vi "AsyncMessageCore.vi"(6 "Timeout (ms)":i32=-1, 7 "Collect Response?":bool, 8 "error in (no error)":errorcluster, 9 "Payload":string, 10 "Command":string, 11 "GRPCClient in":refnum<class "MicronGRPCClient.lvclass">) -> (0 "error out":errorcluster, 3 "GRPCClient out":refnum<class "MicronGRPCClient.lvclass">)   [LabVIEW 2019, in "MicronGRPCClient.lvclass"]
uses:
  MicronGRPCClient.lvclass
  Generated/MicronGRPCGeneratedClient/RPC Messages/micronGrpc_MessageRequest.ctl
  Typedefs/AsyncMessageRequest.ctl
  Typedefs/gRPCDetails.ctl
  <vilib>/gRPC/LabVIEW gRPC Library/Shared/grpcId.ctl
  MicronGRPCClient.lvclass/MicronGRPCClient.ctl
  <vilib>/SLL Toolkit/SLL Queued State Machine/Queue Driver/Enqueue an Item to Queue.vi
  Generated/MicronGRPCGeneratedClient/MicronGRPCGeneratedClient.lvlib
  <vilib>/gRPC/LabVIEW gRPC Library/grpc-lvsupport-release.lvlib
  <vilib>/SLL Toolkit/SLL Queued State Machine/SLL QSM.lvlib
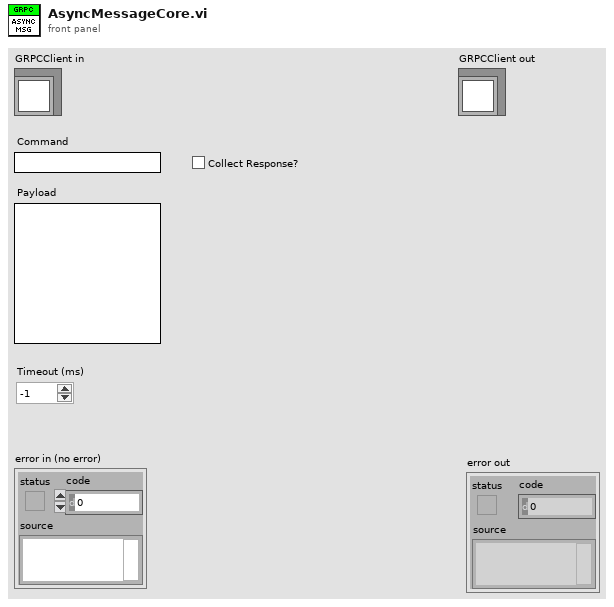
[diagram p1: front panel]
types:
  T1 = typedef "MicronGRPCClient.lvclass/AsyncMessageRequest.ctl" = cluster{"gRPC":T2, "Message":T4, "Timeout (ms)":i32, "Collect Response?":bool}
  T2 = typedef "MicronGRPCClient.lvclass/gRPCDetails.ctl" = cluster{"ID":T3, "PackageName":string, "ServiceName":string, "Simulate?":bool, "ConnectionString":string}
  T3 = typedef "grpc-lvsupport-release.lvlib/grpcId.ctl" = u64
  T4 = typedef "MicronGRPCGeneratedClient.lvlib/micronGrpc_MessageRequest.ctl" = cluster{"command":string, "payload":string}
  T5 = typedef "MicronGRPCClient.lvclass/AsyncCluster.ctl" = cluster{"QueueRef":refnum<queue>, "PackageName":string, "ServiceName":string, "gRPC ID":T3, "Simulate?":bool}
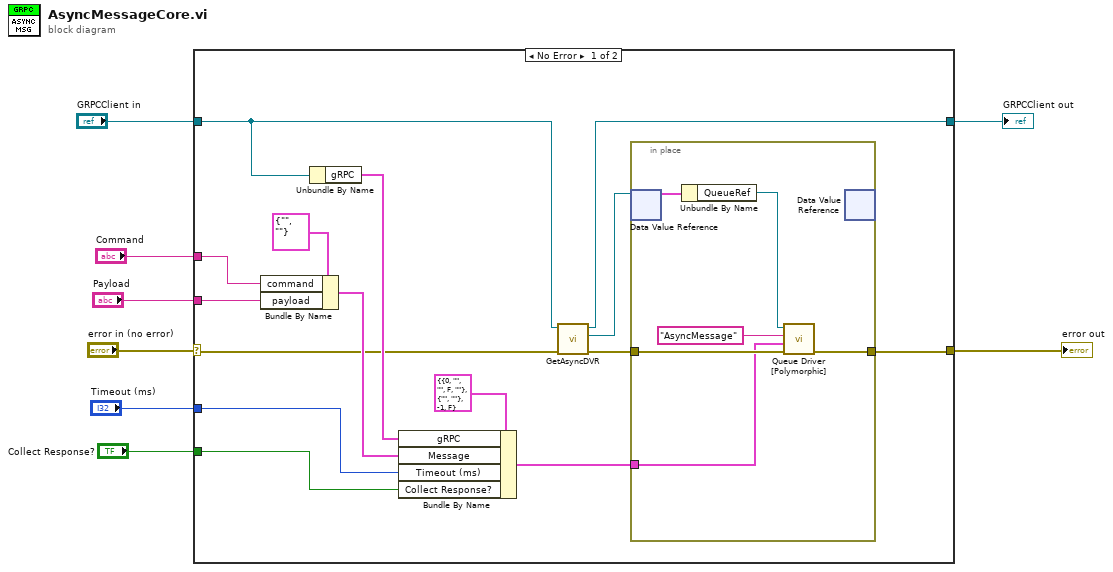
[diagram p0: block diagram]
diagram:
  n1 = case shown="No Error" "error in (no error)" {
    selector: "error in (no error)" -> [w16 w30]
    tunnel: "GRPCClient in" -> [w15 w31]
    tunnel: "Command" -> [w23 _]
    tunnel: "Payload" -> [w22 _]
    tunnel: [w10 w30] -> w4
    tunnel: [w13 w31] -> w3
    tunnel: "Timeout (ms)" -> [w17 _]
    tunnel: "Collect Response?" -> [w9 _]
    frame No Error {
      n2 = Bundle By Name(cluster=T4 {"command"="", "payload"=""} ("Request Data"), "command"=w23, "payload"=w22) -> (w18:T4)
      n3 = Unbundle By Name(w15) -> ("gRPC"=w19:T2)
      n4 = Bundle By Name(cluster=T1 {"gRPC"={"ID"=0, "PackageName"="", "ServiceName"="", "Simulate?"=FALSE, "ConnectionString"=""}, "Message"={"command"="", "payload"=""}, "Timeout (ms)"=-1, "Collect Response?"=FALSE} ("Async"), "gRPC"=w19, "Message"=w18, "Timeout (ms)"=w17, "Collect Response?"=w9) -> (w11:T1)
      n5 = call-dynamic "GetAsyncDVR.vi"("error in (no error)"=w16, "MicronGRPCClient in"=w15) -> ("error out"=w12:errorcluster, "AsyncDVR"=w14:refnum<data-value>, "MicronGRPCClient out"=w13:refnum<class "MicronGRPCClient.lvclass">)  [unwired: 7 in]
      n6 = in-place {
        in-place-border: w12 -> [w28]
        in-place-border: w11 -> [w26]
        in-place-border: [w24] -> w10
        n7 = in-place-dvr #1(w14) -> (w29:T5)  [unwired: 1 out]
        n8 = Unbundle By Name(w29) -> ("QueueRef"=w27:refnum<queue>)
        n9 = call-poly <vilib>:"Queue Driver [Polymorphic].vi"("Error In"=w28, "Data (Optional)"=w26, "Item to Add"="AsyncMessage", "Queue Ref In"=w27) -> ("Error Out"=w24:errorcluster)  [unwired: 6 in, 1 out]
        n10 = in-place-dvr #1() -> ()  [unwired: 1 in, 2 out]
      }
    }
    frame Error {
    }
  }
  "error out" <- w4
  "GRPCClient out" <- w3
